vi "给单元格赋值.vi"(8 "错误输入（无错误）":errorcluster, 9 "新元素/子数组":string, 10 "行列":cluster{"行":i32, "列":i32}, 11 "引用输入":refnum<vi>) -> (0 "错误输出":errorcluster, 3 "引用输出":refnum<vi>)   [LabVIEW 2014, in "表格.lvlib"]
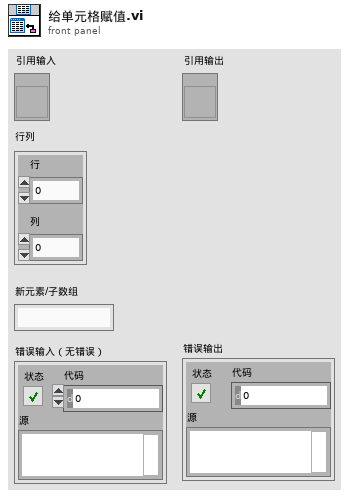
[diagram p1: front panel]
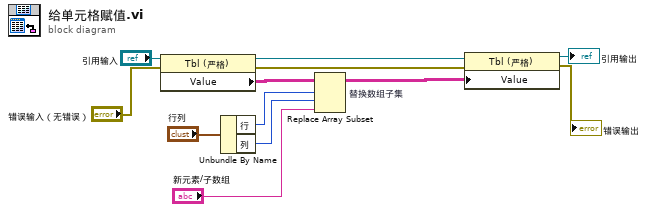
[diagram p0: block diagram]
diagram:
  n1 = property class="Tbl (严格)"(reference="引用输入", error in="错误输入（无错误）") -> (reference out=w12:refnum<vi>, error out=w10:errorcluster, "Value"=w11:string[][])
  n2 = Unbundle By Name("行列") -> ("行"=w8:i32, "列"=w7:i32)
  n3 = Replace Array Subset "替换数组子集"(array=w11, new element="新元素/子数组", index (row)=w8, index (col)=w7) -> (w5:string[][])
  n4 = property class="Tbl (严格)"(reference=w12, error in=w10, "Value"=w5) -> (reference out=→"引用输出":refnum<vi>, error out=→"错误输出":errorcluster)
